vi "Read NowTime.vi"(8 "error in (no error)":errorcluster, 11 "RealWorkActor in":refnum<class "RealWorkActor.lvclass">) -> (0 "error out":errorcluster, 2 "NowTime":timestamp, 3 "RealWorkActor out":refnum<class "RealWorkActor.lvclass">)   [LabVIEW 2014, in "RealWorkActor.lvclass"]
uses:
  RealWorkActor.lvclass
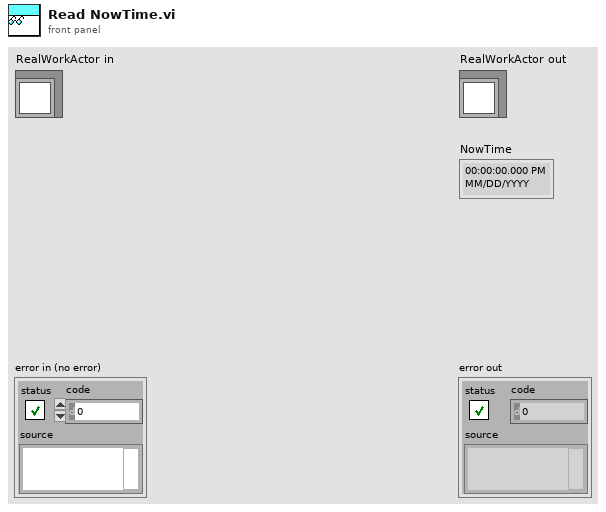
[diagram p1: front panel]
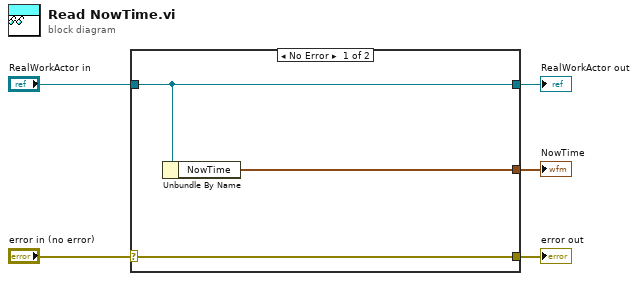
[diagram p0: block diagram]
diagram:
  n1 = case shown="No Error" "error in (no error)" {
    selector: "error in (no error)" -> [w8 w9]
    tunnel: [w8 w9] -> w4
    tunnel: [w7 w10] -> w2
    tunnel: "RealWorkActor in" -> [w7 w10]
    tunnel: [w6 _] -> w1
    frame No Error {
      n2 = Unbundle By Name(w7) -> ("NowTime"=w6:timestamp)
    }
    frame Error {
    }
  }
  "error out" <- w4
  "RealWorkActor out" <- w2
  "NowTime" <- w1
